vi "replace ids.vi"(9 "new ids":string[](array[string]), 10 "old ids":string[](array[string]), 11 "Web Service in":T1) -> (3 "Web Service out":T1)   [LabVIEW 2013]
uses:
  <resource>/Framework/Providers/ws_project_provider/common/Web Service.ctl
  <resource>/Framework/Providers/ws_project_provider/common/Web Service VI.ctl
  <resource>/Framework/Providers/ws_project_provider/common/Web Service VI Type.ctl
  <resource>/Framework/Providers/ws_project_provider/common/Web Service VI Method.ctl
  <resource>/Framework/Providers/ws_project_provider/common/Web Service VI Output Type.ctl
  <resource>/Framework/Providers/ws_project_provider/common/Web Service VI Output Format.ctl
  <resource>/Framework/Providers/ws_project_provider/common/NI Web Service Provider.lvlib
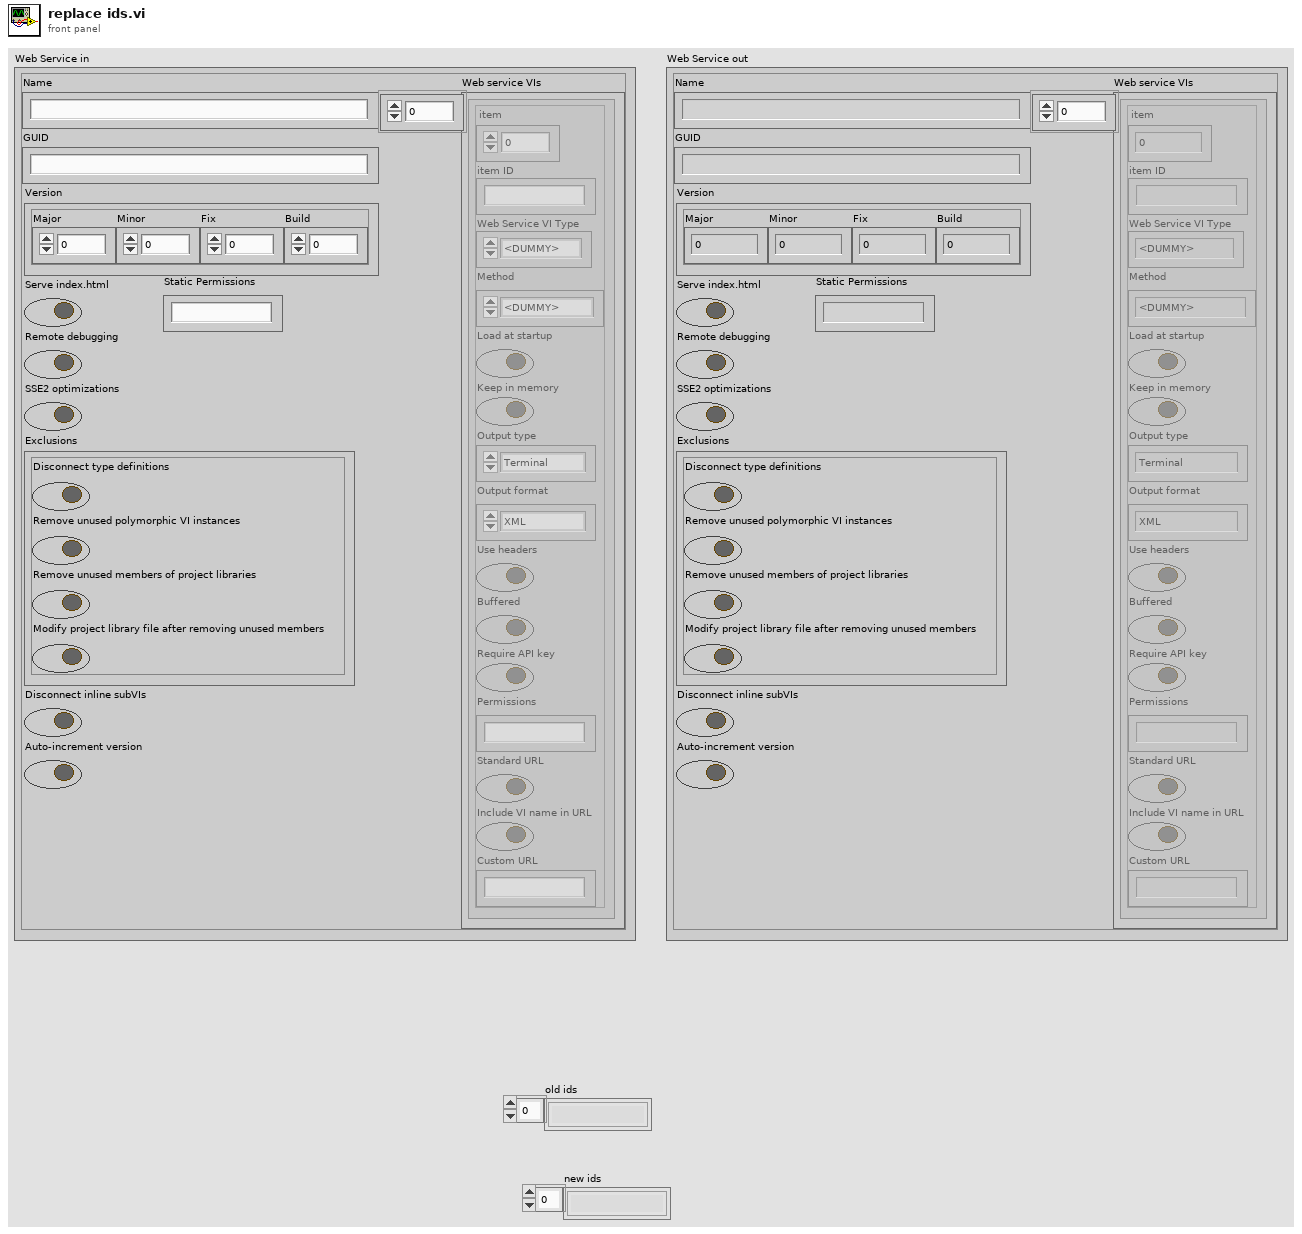
[diagram p1: front panel]
types:
  T1 = typedef "NI Web Service Provider.lvlib/Web Service.ctl" = cluster{"Name":string, "GUID":string, "Version":cluster{"Major":u16, "Minor":u16, "Fix":u16, "Build":u16}, "Serve index.html":bool, "Remote debugging":bool, "SSE2 optimizations":bool, "Exclusions":cluster{"Disconnect type definitions":bool, "Remove unused polymorphic VI instances":bool, "Remove unused members of project libraries":bool, "Modify project library file after removing unused members":bool}, "Disconnect inline subVIs":bool, "Auto-increment version":bool, "Web service VIs":T2[], "Static Permissions":string}
  T2 = typedef "NI Web Service Provider.lvlib/Web Service VI.ctl" = cluster{"item":u64, "item ID":string, "Web Service VI Type":T3, "Method":T4, "Load at startup":bool, "Keep in memory":bool, "Output type":T5, "Output format":T6, "Use headers":bool, "Buffered":bool, "Require API key":bool, "Permissions":string, "Standard URL":bool, "Include VI name in URL":bool, "Custom URL":string}
  T3 = typedef "NI Web Service Provider.lvlib/Web Service VI Type.ctl" = enum16{"<DUMMY>", "Web Method", "Auxiliary", "Internal", "Content"}
  T4 = typedef "NI Web Service Provider.lvlib/Web Service VI Method.ctl" = enum16{"<DUMMY>", "GET", "PUT", "POST", "DELETE", "OPTIONS", "HEAD", "TRACE"}
  T5 = typedef "NI Web Service Provider.lvlib/Web Service VI Output Type.ctl" = enum16{"Terminal", "Stream"}
  T6 = typedef "NI Web Service Provider.lvlib/Web Service VI Output Format.ctl" = enum16{"<DUMMY>", "Text", "XML", "HTML", "JSON"}
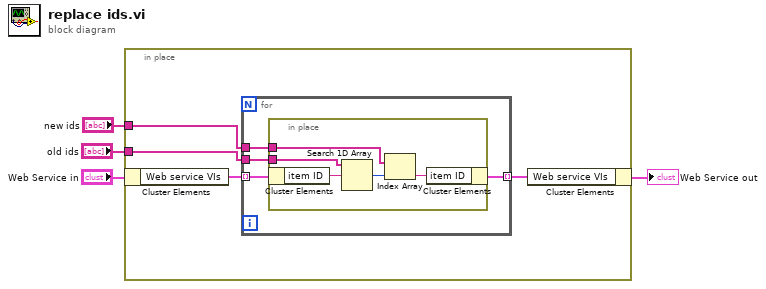
[diagram p0: block diagram]
diagram:
  n1 = in-place {
    in-place-border: "old ids" -> [w6]
    in-place-border: "new ids" -> [w5]
    n2 = in-place-cluster #1("Web Service in") -> ("Web service VIs"=w8:T2[])
    n3 = for {
      tunnel: w8 -> [w12] mode=indexing
      tunnel: [w11] -> w7 mode=indexing
      tunnel: w6 -> [w10]
      tunnel: w5 -> [w9]
      n4 = in-place {
        in-place-border: w10 -> [w16]
        in-place-border: w9 -> [w15]
        n5 = in-place-cluster #2(w12) -> ("item ID"=w17:string)
        n6 = Search 1D Array(1D array=w16, element=w17) -> (index of element=w14:i32)  [unwired: 1 in]
        n7 = Index Array(array=w15, index=w14) -> (element=w13:string)
        n8 = in-place-cluster #2("item ID"=w13) -> (w11:T2)
      }
    }
    n9 = in-place-cluster #1("Web service VIs"=w7) -> (→"Web Service out":T1)
  }
